vi "ConfigureDlg.vi"(8 "error in (no error)":errorcluster, 11 "FunctionBase in":refnum<class "FunctionBase.lvclass">) -> (0 "error out":errorcluster, 2 "Changed":bool, 3 "FunctionBase out":refnum<class "FunctionBase.lvclass">)   [LabVIEW 2018, in "Functions.lvlib" / "FunctionBase.lvclass"]
uses:
  FunctionBase.lvclass
panel:
  in  "btnDone":bool
  # "No configurable Parameters for this Function"
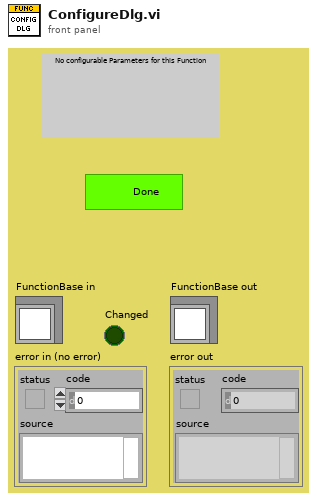
[diagram p1: front panel]
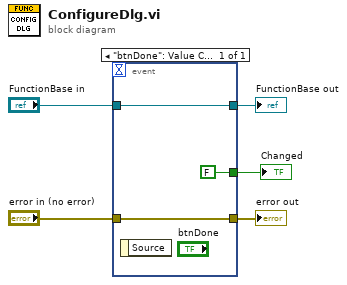
[diagram p0: block diagram]
diagram:
  n1 = event shown="[0] \"btnDone\": Value Change" {
    selector: _ -> [_]
    dyn-events: _ -> [_]
    timeout: _ -> [_]
    tunnel: [w8] -> w4
    tunnel: "error in (no error)" -> [w8]
    tunnel: [FALSE] -> w3
    tunnel: "FunctionBase in" -> [w6]
    tunnel: [w6] -> w1
    event "btnDone": Value Change {
      n2 = event-data() -> ()  [unwired: 1 in, 1 out]
    }
  }
  "error out" <- w4
  "FunctionBase out" <- w1
  "Changed" <- w3
